vi "Save Accelerometer Data SPI.vi"(8 "error in (no error)":errorcluster, 10 "Accelerometer Data Block":T3, 11 "H5refs":T1 {"File ref" format="%.0x"}) -> (0 "error out":errorcluster, 3 "H5refs out":T1 {"File ref" format="%.0x"})   [LabVIEW 2013]
uses:
  I2C/Accelerometer Data Block.ctl
  H5refs.ctl
  <vilib>/addons/h5labview2/base/hid_t.ctl
  h5logger/HDF5 append data (DBL 2D).vi
  h5logger/HDF5 append data (DBL 1D).vi
  h5logger/HDF5 append data (U8 1D).vi
  h5logger/h5logger.lvlib
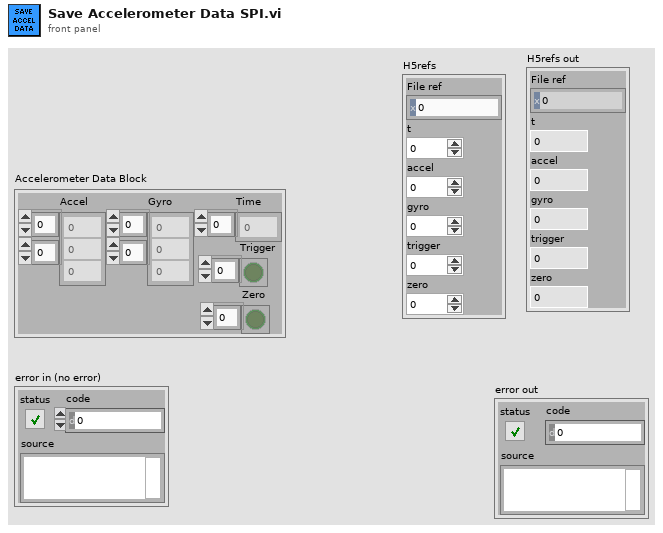
[diagram p1: front panel]
types:
  T1 = typedef "H5refs.ctl" = cluster{"File ref":T2, "t":i32, "accel":i32, "gyro":i32, "trigger":i32, "zero":i32}
  T2 = typedef "hid_t.ctl" = i32
  T3 = typedef "Accelerometer Data Block.ctl" = cluster{"Accel":dbl[][], "Gyro":dbl[][], "Time":u64[], "Trigger":bool[], "Zero":bool[]}
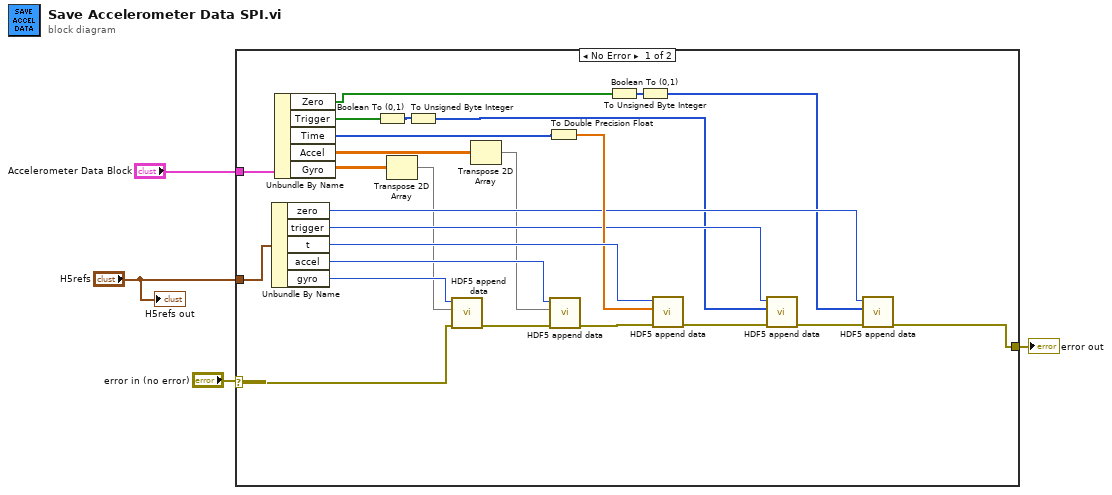
[diagram p0: block diagram]
diagram:
  n1 = case shown="No Error" "error in (no error)" {
    selector: "error in (no error)" -> [w26 w30]
    tunnel: "Accelerometer Data Block" -> [w29 _]
    tunnel: [w16 w30] -> w2
    tunnel: "H5refs" -> [w28 _]
    frame No Error {
      n2 = Unbundle By Name(w28) -> ("zero"=w18:i32, "trigger"=w20:i32, "t"=w22:i32, "accel"=w25:i32, "gyro"=w27:i32)
      n3 = Unbundle By Name(w29) -> ("Zero"=w6:bool[], "Trigger"=w12:bool[], "Time"=w8:u64[], "Accel"=w9:dbl[][], "Gyro"=w10:dbl[][])
      n4 = Boolean To (0,1)(Boolean=w12) -> (0, 1=w11:i16[])
      n5 = Transpose 2D Array(2D array=w10) -> (transposed array=w15:dbl[][])
      n6 = To Unsigned Byte Integer(number=w11) -> (unsigned 8bit integer=w7:u8[])
      n7 = call-poly "HDF5 append data.vi"("error in (no error)"=w26, "data"=w15, "dset in"=w27) -> ("error out"=w24:errorcluster)  [unwired: 7 in, 1 out]
      n8 = Transpose 2D Array(2D array=w9) -> (transposed array=w14:dbl[][])
      n9 = To Double Precision Float(number=w8) -> (double precision float=w21:dbl[])
      n10 = call-poly "HDF5 append data.vi"("error in (no error)"=w24, "data"=w14, "dset in"=w25) -> ("error out"=w23:errorcluster)  [unwired: 7 in, 1 out]
      n11 = Boolean To (0,1)(Boolean=w6) -> (0, 1=w13:i16[])
      n12 = To Unsigned Byte Integer(number=w13) -> (unsigned 8bit integer=w5:u8[])
      n13 = call-poly "HDF5 append data.vi"("error in (no error)"=w23, "data"=w21, "dset in"=w22) -> ("error out"=w19:errorcluster)  [unwired: 7 in, 1 out]
      n14 = call-poly "HDF5 append data.vi"("error in (no error)"=w19, "data"=w7, "dset in"=w20) -> ("error out"=w17:errorcluster)  [unwired: 7 in, 1 out]
      n15 = call-poly "HDF5 append data.vi"("error in (no error)"=w17, "data"=w5, "dset in"=w18) -> ("error out"=w16:errorcluster)  [unwired: 7 in, 1 out]
    }
    frame Error {
    }
  }
  "error out" <- w2
  "H5refs out" <- "H5refs"
